vi "Main FPGA 6-axis Servo.vi"() -> ()   [LabVIEW 2014]
uses:
  <vilib>/Motion/MotorControl/_s/nism.encoder.config.ctl
  <vilib>/Motion/MotorControl/_s/nism.encoder.incremental.config.ctl
  <vilib>/Motion/MotorControl/_s/nism.incremental.indexCriteria.ctl
  <vilib>/Motion/MotorControl/_s/nism.pid.gains.fxp.18.ctl
  <vilib>/Motion/MotorControl/_s/nism.pi.v.outputRange.fxp.6.12.ctl
  <vilib>/Motion/MotorControl/_s/nism.mdo.splineData.ctl
  <vilib>/Motion/MotorControl/_s/nism.splineInterpolation.type.ctl
  <vilib>/Motion/SoftMotion/Synchronization/nism.softmotionScan.timerConfig.ctl
  <vilib>/Platform/TimedLoop/XDataNode/timing_clust.ctl
  <vilib>/Platform/TimedLoop/XDataNode/nitl_modes.ctl
  <vilib>/Platform/TimedLoop/XDataNode/wakeup.ctl
  <vilib>/Motion/MotorControl/_s/nism.digitalInputs.portA.ctl
  <vilib>/rvi/Emulation/niFpgaGetClockAttributes.vi
  <vilib>/rvi/Emulation/niFpgaSctlEmulationGetInTimedLoop.vi
  <vilib>/rvi/Emulation/niFpgaEmulationReportErrorSimple.vi
  Global FPGA 6-axis.vi
  <vilib>/Motion/MotorControl/_s/nism.interpretControlRegister.indexed.vi
  <vilib>/rvi/Emulation/niFpgaProcessEmulError.vi
  <vilib>/Motion/MotorControl/_s/nism.mdo.read.encoder.vi
  <vilib>/Motion/MotorControl/_s/nism.mdo.read.positionLoopSyncData.vi
  <vilib>/Motion/MotorControl/_s/nism.mdo.read.splineData.vi
  <vilib>/Motion/MotorControl/_s/nism.generateStatusRegister.indexed.vi
  <vilib>/rvi/eio/common/nirviEmuTemplateMethod_errors.vi
  <vilib>/rvi/Emulation/niFpgaCriticalErrorInLSC.vi
  <vilib>/Motion/MotorControl/_s/nism.splineInterpolation.fxp.3.index.vi
  <vilib>/Motion/MotorControl/_s/nism.pid.simple.fxp.index.2.vi
  <vilib>/Motion/MotorControl/_s/nism.mdo.handler.indexed.vi
  <vilib>/Motion/MotorControl/_s/nism.digitalFilter.indexed.vi
  <vilib>/Motion/MotorControl/_s/nism.interpretDIOControl.portA.multiple.vi
  <vilib>/Motion/MotorControl/_s/nism.generateDIOStatus.portA.indexed.2.vi
  <vilib>/Motion/SoftMotion/Synchronization/nism.rioScan.generateSyncScan.vi
  <vilib>/Motion/MotorControl/_s/nism.incremental.p.2.vi
  <vilib>/eio/EIONode/EIONode.xnode
  <vilib>/Platform/TimedLoop/XDataNode/XDataNode.xnode
  <vilib>/Motion/MotorControl/NI_SoftMotion_MotorControlIP.lvlib
  <vilib>/Platform/TimedLoop/XDataNode/XDNodeRunTimeDep.lvlib
  <vilib>/Motion/SoftMotion/Synchronization/NI_SoftMotion_Synchronization.lvlib
  <vilib>/rvi/Analysis/measure/butterworth/XNode/niFpgaButterworthFilter.xnode
panel:
  out "Interpolated Position":fxp<+/-,64,32>[](array[numeric])
  in  "Encoder Config (Manual)":T1={"active states"={"line a active high?"=FALSE, "line b active high?"=FALSE, "index active high?"=FALSE}, "index criteria"={"a"=FALSE, "b"=FALSE, "z"=FALSE}, "vel. filter coeffs."=[0, 0, 0]} caption="encoder config"
  in  "Velocity Filter Active?":bool
  in  "Reset Encoder 6":bool caption="reset"
  in  "Reset Encoder 5":bool caption="reset"
  in  "Reset Encoder 4":bool caption="reset"
  in  "Reset Encoder 3":bool caption="reset"
  out "position loop sync":T4
  out "spline":T5 {"spline type" items=["cubic b spline", "catmull-rom spline", "linear"]}
  in  "Reset Encoder 2":bool caption="reset"
  out "Velocity Feedback":i16[](array[numeric])
  out "pos. error":i16[](array[numeric])
  out "pos. error exceeded":bool[](array[boolean])
  in  "calls per sample (vel)":u16=2000 caption="calls per sample"
  in  "Limit Ranges":T7[](array[typedef])=[{"output low"=0.0, "output high"=0.0}, {"output low"=0.0, "output high"=0.0}, {"output low"=0.0, "output high"=0.0}, {"output low"=0.0, "output high"=0.0}, {"output low"=0.0, "output high"=0.0}, {"output low"=0.0, "output high"=0.0}]
  in  "Gains":T8[](array[typedef])=[{"kp"=0.0, "kd"=0.0, "ki"=0.0}, {"kp"=0.0, "kd"=0.0, "ki"=0.0}, {"kp"=0.0, "kd"=0.0, "ki"=0.0}, {"kp"=0.0, "kd"=0.0, "ki"=0.0}, {"kp"=0.0, "kd"=0.0, "ki"=0.0}, {"kp"=0.0, "kd"=0.0, "ki"=0.0}]
  out "AO Check":fxp<+/-,20,5>[](array[numeric])
  in  "AO Manual":fxp<+/-,20,5>[](array[numeric])=[0.0, 0.0, 0.0, 0.0, 0.0, 0.0]
  out "Position Feedback":i32[](array[numeric])
  in  "Reset Encoder 1":bool caption="reset"
  out "corrected period":u16
  in  "AO Disabled?":bool
  out "PID loop time (ticks)":u32
  in  "AO Override?":bool
  in  "position error limit":i16=10000
  in  "Encoder filter value (us) Manual":u16=10
  out "encoder config":T1
  out "Home Limits":bool[](array[boolean])
  out "Fwd Limits":bool[](array[boolean])
  out "Rev Limits":bool[](array[boolean])
  out "Drive Enable":bool[](array[boolean])
  in  "Enable value":bool
  in  "Drive Enable override?":bool
  in  "Sync Value":bool
  in  "Sync Enable override?":bool
  out "Sync is Fault":bool
  out "Sync is Locked":bool
  # "Synchronization Loop"
  # "Control Status Loop"
  # "Notes: \n1. This VI provides the communication interface between the NI SoftMotion Engine and the LabVIEW FPGA Module. You must compile this VI for a specific FPGA target before use. After compiling, run the VI before running any of the Express VI examples. For information on moving this example to another FPGA target, refer to ni.com/info and enter info code fpgaex.\n\n2. Only use the Reset Axis button if you are unable to communicate with the axis by any other means. This button resets the device state machine and other VIs to a known state. After resetting the axis, switch the NI Scan Engine from Active Mode to Configuration Mode, then back to Active Mode, before attempting to enable the axis."
  # "(These two buttons \nare for testing\npurposes.)"
  # "(These two buttons \nare for testing\npurposes.)"
  # "Position/PID Loop"
  # "Parameter Check"
  # "AO Debug"
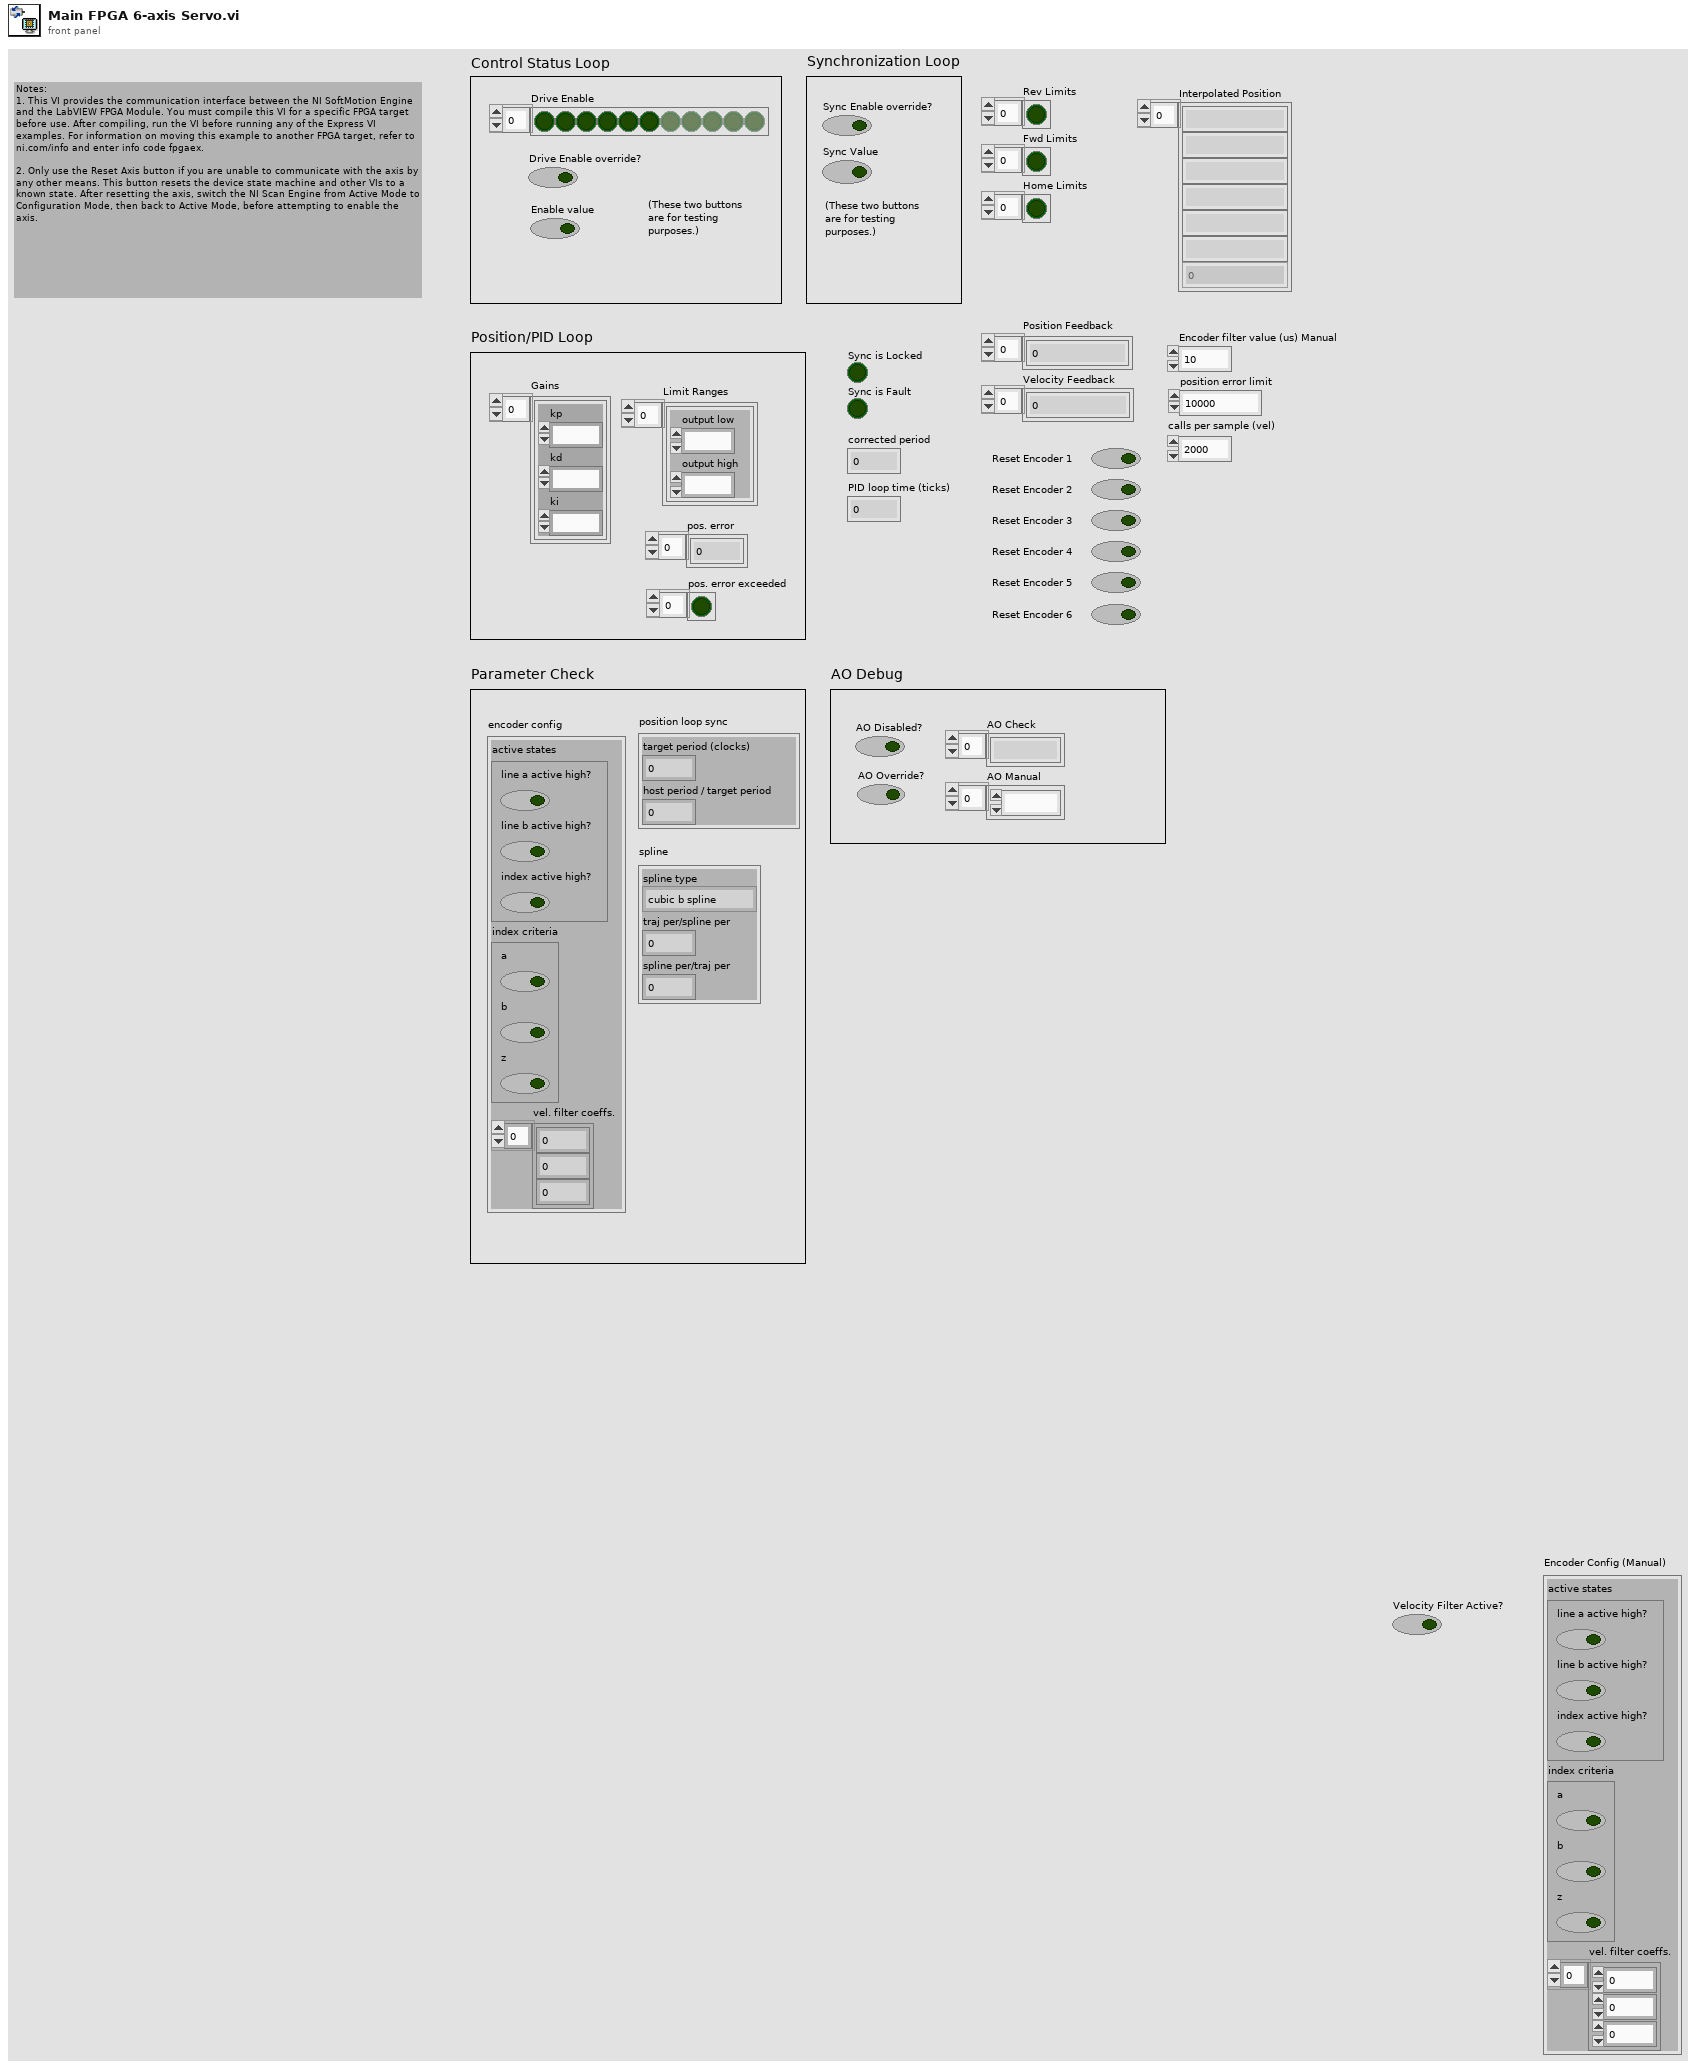
[diagram p1: front panel]
types:
  T1 = typedef "NI_SoftMotion_MotorControlIP.lvlib/nism.encoder.config.ctl" = cluster{"active states":T2, "index criteria":T3, "vel. filter coeffs.":i32[]}
  T2 = typedef "NI_SoftMotion_MotorControlIP.lvlib/nism.encoder.incremental.config.ctl" = cluster{"line a active high?":bool, "line b active high?":bool, "index active high?":bool}
  T3 = typedef "NI_SoftMotion_MotorControlIP.lvlib/nism.incremental.indexCriteria.ctl" = cluster{"a":bool, "b":bool, "z":bool}
  T4 = typedef "NI_SoftMotion_Synchronization.lvlib/nism.softmotionScan.timerConfig.ctl" = cluster{"target period (clocks)":u16, "host period / target period":u16}
  T5 = typedef "NI_SoftMotion_MotorControlIP.lvlib/nism.mdo.splineData.ctl" = cluster{"spline type":T6, "traj per/spline per":u16, "spline per/traj per":fxp<+,32,0>}
  T6 = typedef "NI_SoftMotion_MotorControlIP.lvlib/nism.splineInterpolation.type.ctl" = u16
  T7 = typedef "NI_SoftMotion_MotorControlIP.lvlib/nism.pi.v.outputRange.fxp.6.12.ctl" = cluster{"output low":fxp<+/-,18,6>, "output high":fxp<+/-,18,6>}
  T8 = typedef "NI_SoftMotion_MotorControlIP.lvlib/nism.pid.gains.fxp.18.ctl" = cluster{"kp":fxp<+,18,7>, "kd":fxp<+,18,7>, "ki":fxp<+,18,0>}
  T9 = typedef "XDNodeRunTimeDep.lvlib/timing_clust.ctl" = cluster{"Expected End [f-1]":u64, "Actual End [f-1]":u64, "Finished Late? [f-1]":bool, "Expected End [i-1]":u64, "Actual End [i-1]":u64, "Finished Late? [i-1]":bool, "Expected Start [i]":u64, "Actual Start [i]":u64, "Expected Start [f]":u64, "Actual Start [f]":u64, "Source Name":string, "Structure Name":string, "Period":i64, "Deadline":i64, "Offset":i64, "Start":i64, "Priority":i32, "Timeout":i32, "Mode":T10, "Wakeup Reason":T11, "Error":errorcluster, "Source Type":string, "Secondary Source Type":string, "Global End Time":u64, "Global Start Time":u64, "Frame Duration":u64, "Iteration Duration":u64, "Assigned CPU":i32, "I/O Scan Engine Mode":u32}
  T10 = typedef "XDNodeRunTimeDep.lvlib/nitl_modes.ctl" = enum32{"No Change", "Process missed periods, maintain original phase", "Discard missed periods, maintain original phase", "Process missed periods, ignore original phase", "Discard missed periods, ignore original phase"}
  T11 = typedef "XDNodeRunTimeDep.lvlib/wakeup.ctl" = enum32{"Normal", "Aborted", "Asynchronous wakeup", "Timing source error", "Timed loop error", "Timeout"}
  T12 = typedef "NI_SoftMotion_MotorControlIP.lvlib/nism.digitalInputs.portA.ctl" = cluster{"reverse limit":bool, "forward limit":bool, "home switch":bool, "digital input 0":bool, "digital input 1":bool, "digital input 2":bool, "digital input 3":bool}
  T13 = typedef "NI_SoftMotion_MotorControlIP.lvlib/nism.dio.portA.config.2.ctl" = cluster{"digital filter (us)":u16[], "safe state":T14[]}
  T14 = typedef "nism.safeStates.ctl" = enum8{"Low", "High", "No Change"}
  T15 = typedef "NI_SoftMotion_Synchronization.lvlib/nism.softmotionScan.timerControl.ctl" = cluster{"sm scan":bool, "sm scan count":u32, "sm scan enabled":bool}
  T16 = typedef "NI_SoftMotion_MotorControlIP.lvlib/nism.interpretControlRegister.stateTransition.ctl" = enum8{"Invalid", "Start --> Initializing", "Initializing --> Disabled", "Disabled --> Ready To Switch On", "Ready To Switch On --> Switched On", "Ready To Switch On --> Disable", "Switched On --> Operation Enable", "Switched On --> Ready To Switch On", "Switched On --> Disabled", "Operation Enable --> Switched On", "Operation Enable --> Ready To Switch On", "Operation Enable --> Disabled", "Fault --> Disabled", "Any --> Fault", "None"}
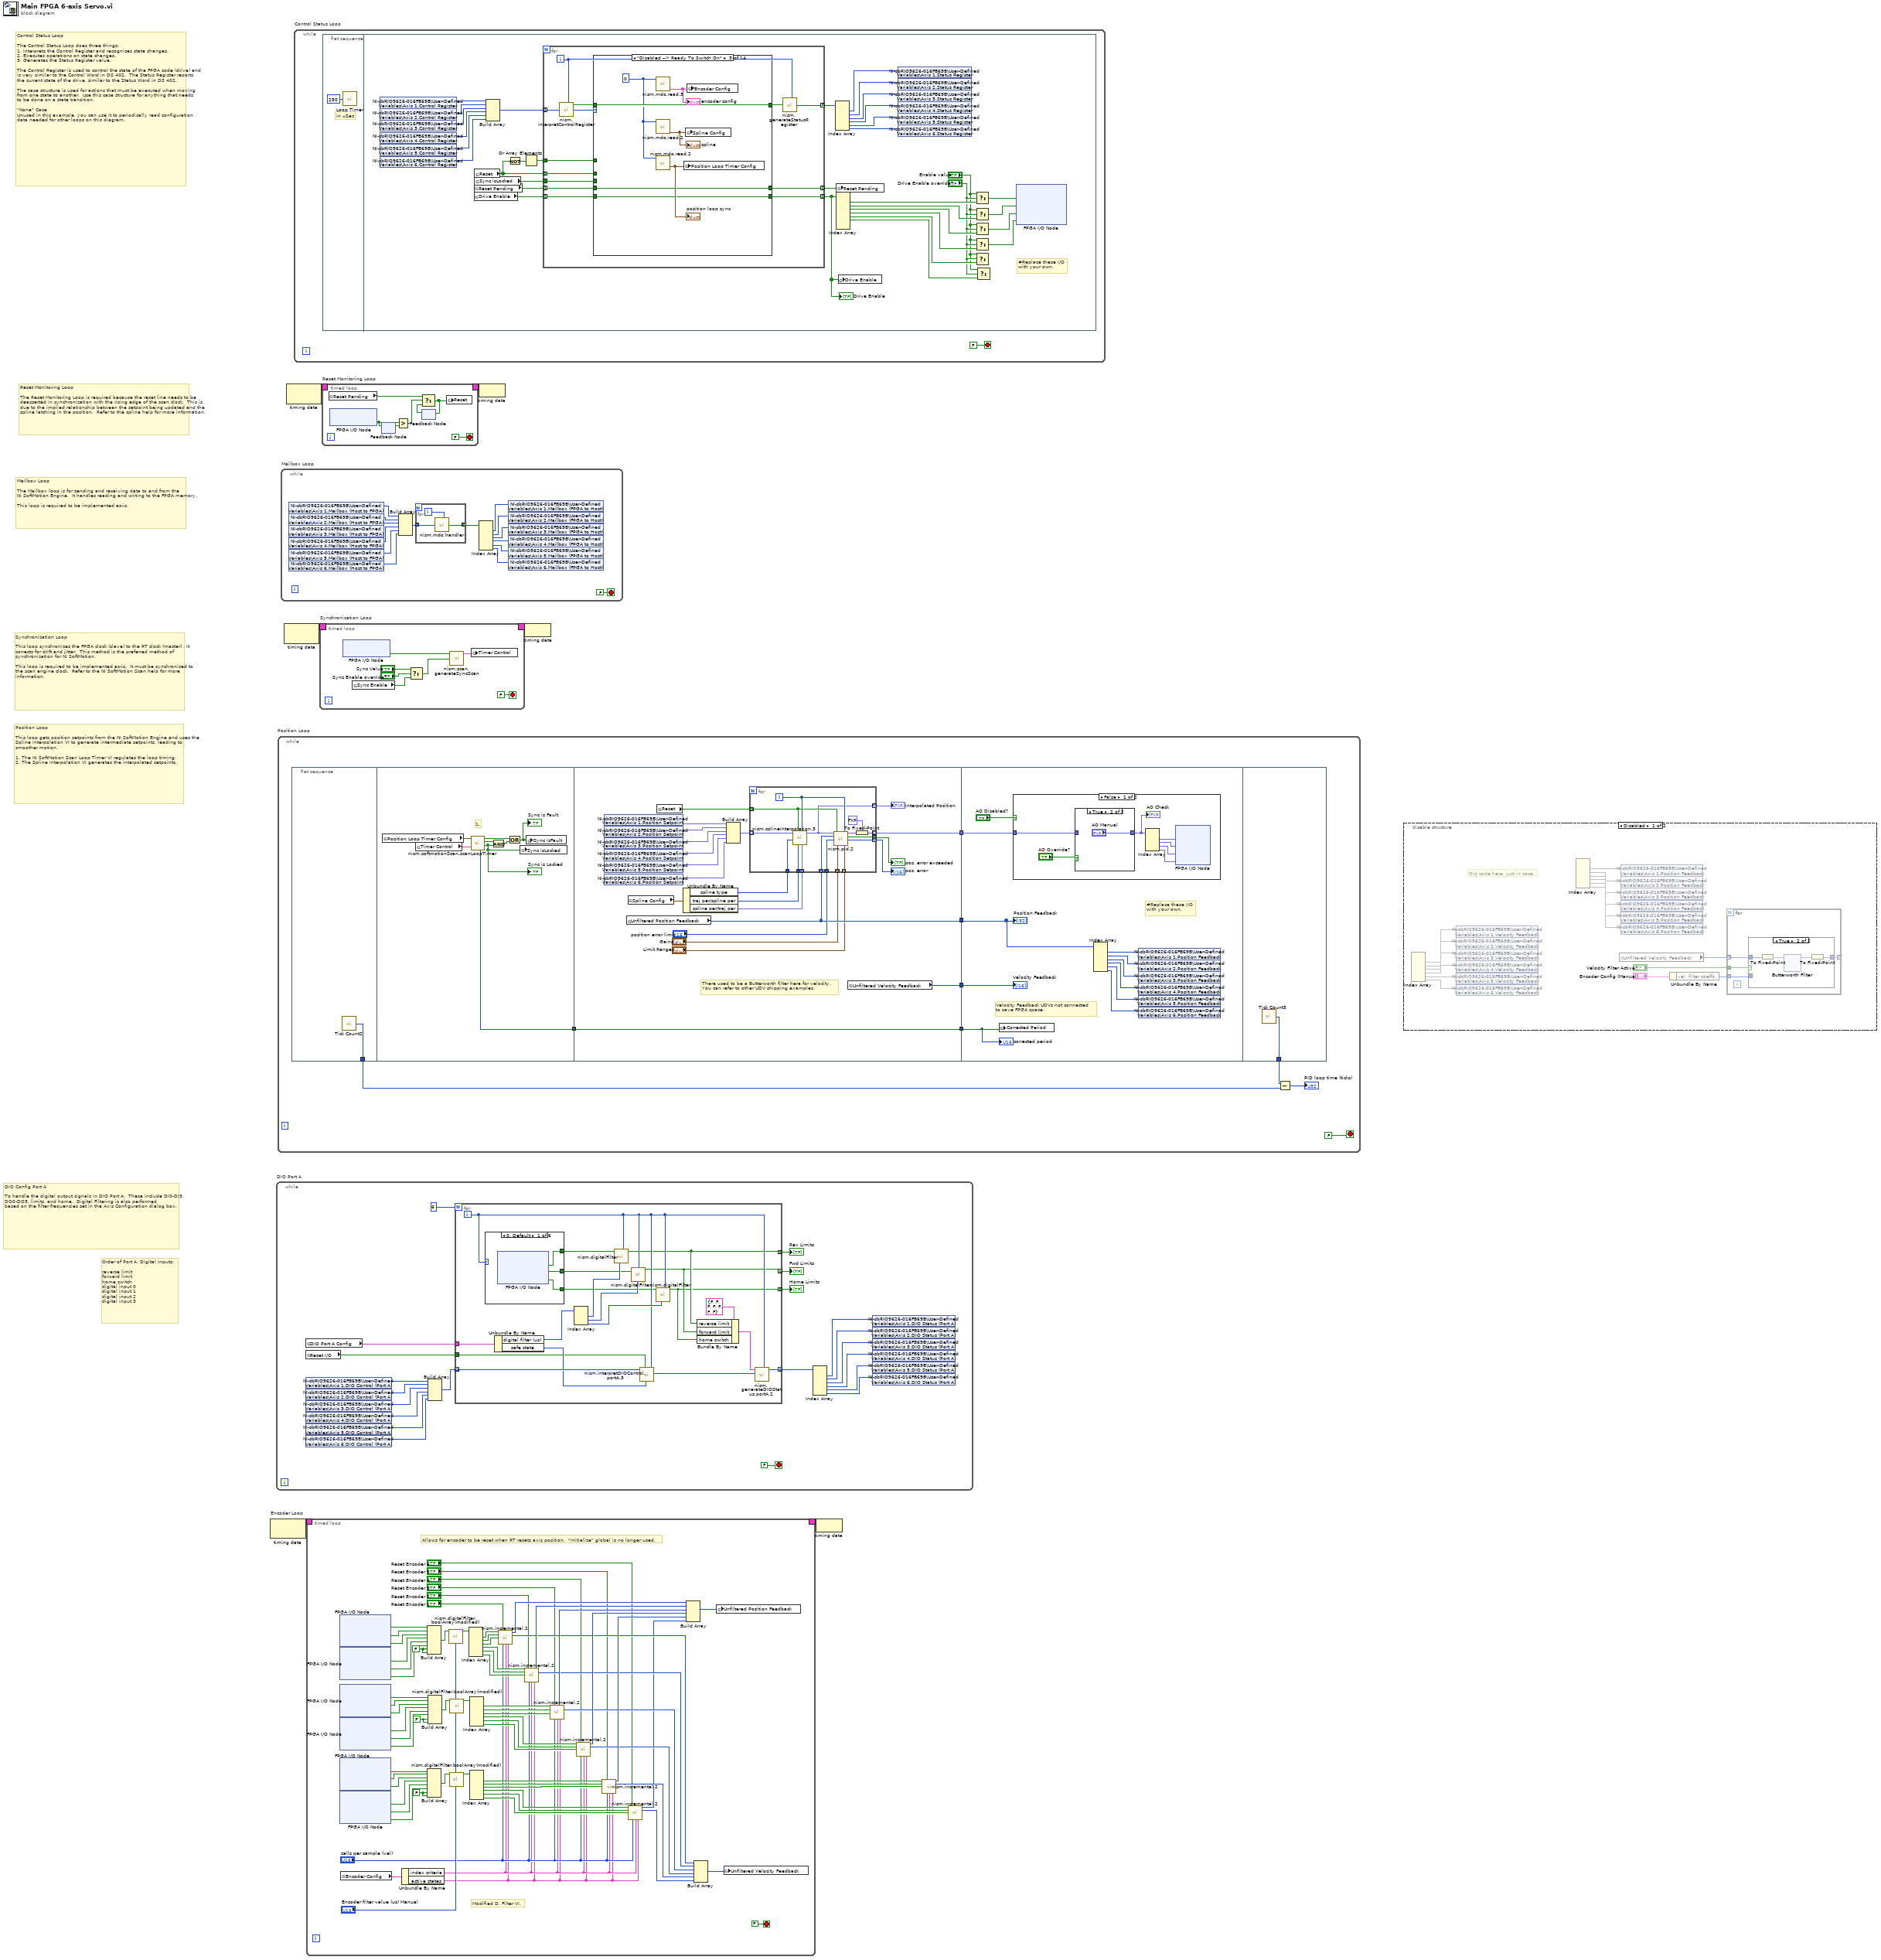
[diagram p0: block diagram]
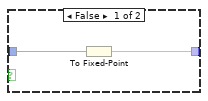
[diagram p2: hidden frame]
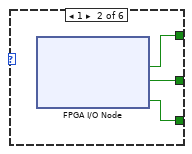
[diagram p4: hidden frame]
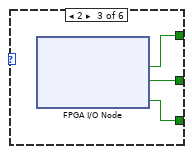
[diagram p5: hidden frame]
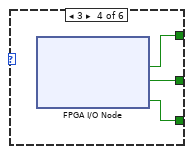
[diagram p6: hidden frame]
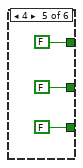
[diagram p7: hidden frame]
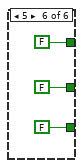
[diagram p8: hidden frame]
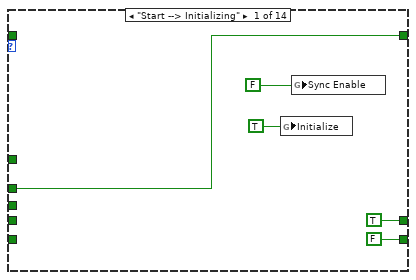
[diagram p11: hidden frame]
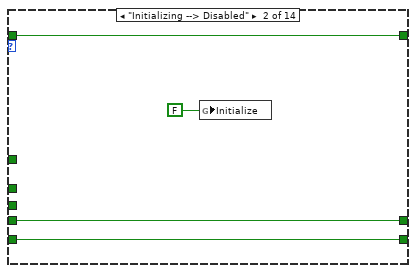
[diagram p12: hidden frame]
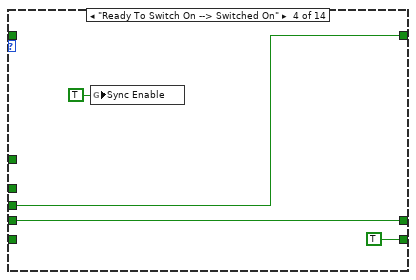
[diagram p13: hidden frame]
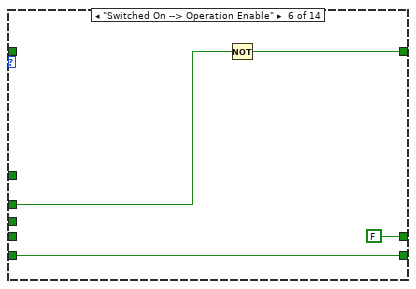
[diagram p15: hidden frame]
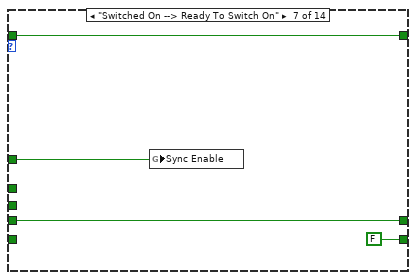
[diagram p16: hidden frame]
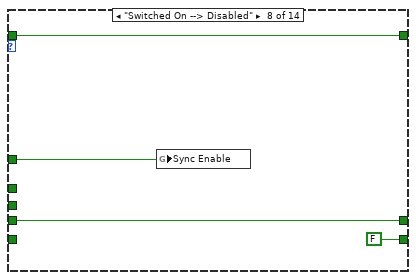
[diagram p17: hidden frame]
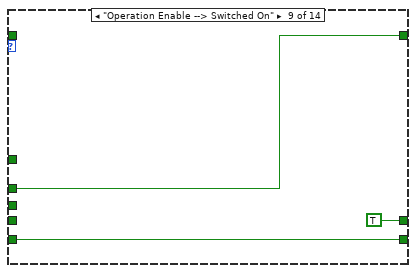
[diagram p18: hidden frame]
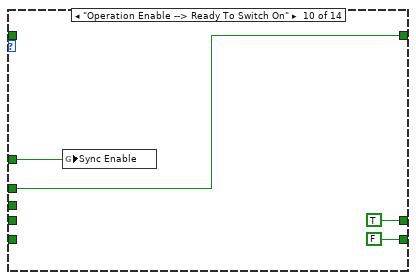
[diagram p19: hidden frame]
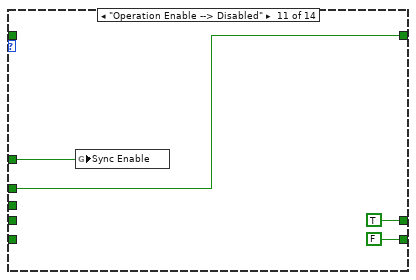
[diagram p20: hidden frame]
diagram:
  # "DIO Config Port A\n\nTo handle the digital output signals in DIO Port A.  These include DI0-DI3, DO0-DO3, limits, and home.  Digital Filtering is also performed\nbased on the filter frequencies set in the Axis Configuration dialog box."
  # "Order of Port A, Digital Inputs:\n\nreverse limit\nforward limit\nhome switch\ndigital input 0\ndigital input 1\ndigital input 2\ndigital input 3"
  # "Position Loop\n\nThis loop gets position setpoints from the NI SoftMotion Engine and uses the Spline Interpolation VI to generate intermediate setpoints, leading to smoother motion.\n\n1. The NI SoftMotion Scan Loop Timer VI regulates the loop timing. \n2. The Spline Interpolation VI generates the interpolated setpoints."
  # "Synchronization Loop\n\nThis loop synchronizes the FPGA clock (slave) to the RT clock (master).  It corrects for drift and jitter.  This method is the preferred method of synchronization for NI SoftMotion.\n\nThis loop is required to be implemented as-is.  It must be synchronized to the scan engine clock.  Refer to the NI SoftMotion Scan help for more information."
  # "Mailbox Loop\n\nThe Mailbox loop is for sending and receiving data to and from the \nNI SoftMotion Engine.  It handles reading and writing to the FPGA memory.\n\nThis loop is required to be implemented as-is."
  # "Reset Monitoring Loop\n\nThe Reset Monitoring Loop is required because the reset line needs to be deasserted in synchronization with the rising edge of the scan clock.  This is due to the implied relationship between the setpoint being updated and the spline latching in the position.  Refer to the spline help for more information."
  # "Control Status Loop\n\nThe Control Status Loop does three things:\n1. Interprets the Control Register and recognizes state changes.\n2. Executes operations on state changes.\n3. Generates the Status Register value.\n\nThe Control Register is used to control the state of the FPGA code (drive) and is very similar to the Control Word in DS 402.  The Status Register reports the current state of the drive, similar to the Status Word in DS 402.\n\nThe case structure is used for actions that must be executed when moving from one state to another.  Use this case structure for anything that needs to be done on a state transition.\n\n\"None\" Case\nUnused in this example, you can use it to periodically read configuration data needed for other loops on this diagram."
  n1 = node-c288() -> (w2:T9)  [unwired: 1 in]
  n2 = while "DIO Port A" {
    stop <- FALSE stop-if-true
    n3 = global read "Global FPGA 6-axis.vi" "DIO Port A Config"() -> (w26:T13)
    n4 = global read "Global FPGA 6-axis.vi" "Reset I/O"() -> (w25:bool)
    n5 = shared-variable "NI-sbRIO9626-016FB69B\\User-Defined Variables\\Axis 1.DIO Control (Port A)"() -> (w23:u32)  [unwired: 1 in, 1 out]
    n6 = shared-variable "NI-sbRIO9626-016FB69B\\User-Defined Variables\\Axis 2.DIO Control (Port A)"() -> (w22:u32)  [unwired: 1 in, 1 out]
    n7 = shared-variable "NI-sbRIO9626-016FB69B\\User-Defined Variables\\Axis 3.DIO Control (Port A)"() -> (w21:u32)  [unwired: 1 in, 1 out]
    n8 = shared-variable "NI-sbRIO9626-016FB69B\\User-Defined Variables\\Axis 4.DIO Control (Port A)"() -> (w20:u32)  [unwired: 1 in, 1 out]
    n9 = shared-variable "NI-sbRIO9626-016FB69B\\User-Defined Variables\\Axis 5.DIO Control (Port A)"() -> (w19:u32)  [unwired: 1 in, 1 out]
    n10 = shared-variable "NI-sbRIO9626-016FB69B\\User-Defined Variables\\Axis 6.DIO Control (Port A)"() -> (w8:u32)  [unwired: 1 in, 1 out]
    n11 = Build Array(w23, w22, w21, w20, w19, w8) -> (w18:u32[])
    n12 = for {
      N: 6 -> [_]
      tunnel: [w45] -> w12 mode=indexing
      tunnel: w18 -> [w44] mode=indexing
      tunnel: w26 -> [w41]
      tunnel: w25 -> [w39]
      tunnel: [w30] -> w11 mode=indexing
      tunnel: [w29] -> w10 mode=indexing
      tunnel: [w28] -> w9 mode=indexing
      i -> [w34]
      n13 = case shown="0, Default" w34 {
        tunnel: [w49 w52 w55 w58 FALSE ("RMC/DIO44") FALSE ("RMC/DIO44")] -> w33
        tunnel: [w47 w50 w53 w56 FALSE ("RMC/DIO61") FALSE ("RMC/DIO61")] -> w32
        tunnel: [w48 w51 w54 w57 FALSE ("RMC/DIO77") FALSE ("RMC/DIO77")] -> w31
        frame 0, Default {
          n14 = xnode "FPGA I/O Node"() -> ("RMC/DIO29"=w49:bool, "RMC/DIO93"=w48:bool, "RMC/DIO11"=w47:bool)  [unwired: 3 in, 3 out]
        }
        frame 1 {
          n15 = xnode "FPGA I/O Node"() -> ("RMC/DIO44"=w52:bool, "RMC/DIO77"=w51:bool, "RMC/DIO61"=w50:bool)  [unwired: 3 in, 3 out]
        }
        frame 2 {
          n16 = xnode "FPGA I/O Node"() -> ("RMC/DIO31"=w55:bool, "RMC/DIO95"=w54:bool, "RMC/DIO13"=w53:bool)  [unwired: 3 in, 3 out]
        }
        frame 3 {
          n17 = xnode "FPGA I/O Node"() -> ("RMC/DIO47"=w58:bool, "RMC/DIO46"=w57:bool, "RMC/DIO79"=w56:bool)  [unwired: 3 in, 3 out]
        }
        frame 4 {
        }
        frame 5 {
        }
      }
      n18 = Unbundle By Name(w41) -> ("digital filter (us)"=w35:u16[], "safe state"=w40:T14[])
      n19 = Index Array(array=w35) -> (element #1=w36:u16, element #2=w37:u16, element #3=w38:u16)  [unwired: 3 in]
      n20 = call-poly <vilib>:"nism.digitalFilter.vi"("index"=w34, "filter value (us)"=w36, "input signal"=w33) -> ("output signal"=w30:bool)  [unwired: 8 in]
      n21 = call-poly <vilib>:"nism.digitalFilter.vi"("index"=w34, "filter value (us)"=w37, "input signal"=w31) -> ("output signal"=w29:bool)  [unwired: 8 in]
      n22 = call-poly <vilib>:"nism.interpretDIOControl.portA.3.vi"("index"=w34, "safe state"=w40, "reset"=w39, "dio control(port a)"=w44) -> ("reset latches"=w46:u8)  [unwired: 6 in, 1 out]
      n23 = call-poly <vilib>:"nism.digitalFilter.vi"("index"=w34, "filter value (us)"=w38, "input signal"=w32) -> ("output signal"=w28:bool)  [unwired: 8 in]
      n24 = Bundle By Name(cluster=T12 {"reverse limit"=FALSE, "forward limit"=FALSE, "home switch"=FALSE, "digital input 0"=FALSE, "digital input 1"=FALSE, "digital input 2"=FALSE, "digital input 3"=FALSE} ("$(driveInterface.digitalInputs.shortName)"), "reverse limit"=w30, "forward limit"=w29, "home switch"=w28) -> (w42:T12)
      n25 = call-poly <vilib>:"nism.generateDIOStatus.portA.2.vi"("index"=w34, "reset latches"=w46, "digital inputs"=w42) -> ("dio status(port a)"=w45:u32)  [unwired: 8 in]
    }
    "Rev Limits" <- w11
    "Fwd Limits" <- w10
    "Home Limits" <- w9
    n26 = Index Array(array=w12) -> (element #1=w17:u32, element #2=w16:u32, element #3=w15:u32, element #4=w14:u32, element #5=w13:u32, element #6=w7:u32)  [unwired: 6 in]
    n27 = shared-variable "NI-sbRIO9626-016FB69B\\User-Defined Variables\\Axis 1.DIO Status (Port A)"(w17) -> ()  [unwired: 1 in, 1 out]
    n28 = shared-variable "NI-sbRIO9626-016FB69B\\User-Defined Variables\\Axis 2.DIO Status (Port A)"(w16) -> ()  [unwired: 1 in, 1 out]
    n29 = shared-variable "NI-sbRIO9626-016FB69B\\User-Defined Variables\\Axis 3.DIO Status (Port A)"(w15) -> ()  [unwired: 1 in, 1 out]
    n30 = shared-variable "NI-sbRIO9626-016FB69B\\User-Defined Variables\\Axis 4.DIO Status (Port A)"(w14) -> ()  [unwired: 1 in, 1 out]
    n31 = shared-variable "NI-sbRIO9626-016FB69B\\User-Defined Variables\\Axis 5.DIO Status (Port A)"(w13) -> ()  [unwired: 1 in, 1 out]
    n32 = shared-variable "NI-sbRIO9626-016FB69B\\User-Defined Variables\\Axis 6.DIO Status (Port A)"(w7) -> ()  [unwired: 1 in, 1 out]
  }
  n33 = while "Position Loop" {
    stop <- FALSE stop-if-true
    n34 = flat-sequence {
      tunnel: [w74] -> w68
      tunnel: [w75] -> w71
      tunnel: [w100] -> w72
      tunnel: w71 -> [w100]
      tunnel: [w90] -> w70
      tunnel: [w94] -> w66
      tunnel: [w84] -> w65
      tunnel: w72 -> [w131]
      tunnel: w70 -> [w121]
      tunnel: w66 -> [w130]
      tunnel: w65 -> [w128]
      tunnel: [w141] -> w69
      frame #0 {
        n35 = call "Tick Count2"() -> ("Tick Count(Ticks)"=w74:u32)
      }
      frame #1 {
        # "1."
        n36 = global read "Global FPGA 6-axis.vi" "Position Loop Timer Config"() -> (w77:T4)
        n37 = global read "Global FPGA 6-axis.vi" "Timer Control"() -> (w76:T15)
        n38 = call <vilib>:"nism.softmotionScan.scanLoopTimer.vi"("timer control"=w76, "timer config"=w77) -> ("scan running?"=w79:bool, "finished late?"=w81:bool, "fault occurred?"=w82:bool, "corrected period"=w75:u16)  [unwired: 5 in, 1 out]
        "Sync is Locked" <- w79
        n39 = Compound Arithmetic op=AND(w81, w79) -> (w80:bool)
        n40 = Compound Arithmetic op=OR(w82, w80) -> (w78:bool)
        "Sync is Fault" <- w78
        n41 = global write "Global FPGA 6-axis.vi" "Sync isLocked"(w79) -> ()
        n42 = global write "Global FPGA 6-axis.vi" "Sync isFault"(w78) -> ()
      }
      frame #2 {
        # "There used to be a Butterworth filter here for velocity.  \nYou can refer to other UDV shipping examples."
        n43 = shared-variable "NI-sbRIO9626-016FB69B\\User-Defined Variables\\Axis 1.Position Setpoint"() -> (w95:fxp<+/-,64,32>)  [unwired: 1 in, 1 out]
        n44 = shared-variable "NI-sbRIO9626-016FB69B\\User-Defined Variables\\Axis 2.Position Setpoint"() -> (w99:fxp<+/-,64,32>)  [unwired: 1 in, 1 out]
        n45 = shared-variable "NI-sbRIO9626-016FB69B\\User-Defined Variables\\Axis 3.Position Setpoint"() -> (w98:fxp<+/-,64,32>)  [unwired: 1 in, 1 out]
        n46 = shared-variable "NI-sbRIO9626-016FB69B\\User-Defined Variables\\Axis 4.Position Setpoint"() -> (w97:fxp<+/-,64,32>)  [unwired: 1 in, 1 out]
        n47 = shared-variable "NI-sbRIO9626-016FB69B\\User-Defined Variables\\Axis 5.Position Setpoint"() -> (w96:fxp<+/-,64,32>)  [unwired: 1 in, 1 out]
        n48 = shared-variable "NI-sbRIO9626-016FB69B\\User-Defined Variables\\Axis 6.Position Setpoint"() -> (w87:fxp<+/-,64,32>)  [unwired: 1 in, 1 out]
        n49 = global read "Global FPGA 6-axis.vi" "Unfiltered Position Feedback"() -> (w90:i32[])
        n50 = global read "Global FPGA 6-axis.vi" "Spline Config"() -> (w101:T5)
        n51 = global read "Global FPGA 6-axis.vi" "Reset"() -> (w92:bool[])
        n52 = Unbundle By Name(w101) -> ("spline type"=w104:T6, "traj per/spline per"=w103:u16, "spline per/traj per"=w102:fxp<+,32,0>)
        n53 = Build Array(w95, w99, w98, w97, w96, w87) -> (w93:fxp<+/-,64,32>[])
        n54 = for {
          tunnel: w104 -> [w120]
          tunnel: w103 -> [w119]
          tunnel: w102 -> [w118]
          tunnel: "Limit Ranges" -> [w117] mode=indexing
          tunnel: [w107] -> w94 mode=indexing
          tunnel: w93 -> [w116] mode=indexing
          tunnel: w92 -> [w114] mode=indexing
          tunnel: w90 -> [w113] mode=indexing
          tunnel: "position error limit" -> [w112]
          tunnel: [w111] -> w86 mode=indexing
          tunnel: [w110] -> w85 mode=indexing
          tunnel: "Gains" -> [w106] mode=indexing
          tunnel: [w105] -> w83 mode=indexing
          i -> [w115]
          n55 = call-poly <vilib>:"nism.splineInterpolation.3.vi"("1 / calls per sample"=w118, "index"=w115, "calls per sample"=w119, "reset"=w114, "spline type"=w120, "x"=w116) -> ("xi"=w105:fxp<+/-,64,32>)  [unwired: 4 in, 1 out]
          n56 = call-poly <vilib>:"nism.pid.2.vi"("position setpoint"=w105, "position feedback"=w113, "position error limit"=w112, "reset"=w114, "gains"=w106, "index"=w115, "output range"=w117) -> ("current setpoint"=w108:fxp<+/-,18,6>, "pos. error exceeded"=w111:bool, "position error"=w110:i16)  [unwired: 10 in]
          n57 = To Fixed-Point(fixed-point type=fxp<+/-,20,5> 0.0 ("AO 1"), number=w108) -> (fixed-point=w107:fxp<+/-,20,5>)
        }
        "pos. error exceeded" <- w86
        "pos. error" <- w85
        "Interpolated Position" <- w83
        n58 = global read "Global FPGA 6-axis.vi" "Unfiltered Velocity Feedback"() -> (w84:i16[])
      }
      frame #3 {
        # "Velocity Feedback UDVs not connected\nto save FPGA space."
        # "#Replace these I/O\nwith your own."
        n59 = global write "Global FPGA 6-axis.vi" "Corrected Period"(w131) -> ()
        n60 = case shown="False" "AO Disabled?" {
          tunnel: w130 -> [w137 _]
          frame False {
            n61 = case shown="True" "AO Override?" {
              tunnel: w137 -> [w139 _]
              tunnel: [w139 "AO Manual"] -> w136
              frame False {
              }
              frame True {
              }
            }
            "AO Check" <- w136
            n62 = Index Array(array=w136) -> (element #1=w135:fxp<+/-,20,5>, element #2=w134:fxp<+/-,20,5>, element #3=w133:fxp<+/-,20,5>, element #4=w132:fxp<+/-,20,5>)  [unwired: 4 in]
            n63 = xnode "FPGA I/O Node"("AO0"=w135, "AO1"=w134, "AO2"=w133, "AO3"=w132) -> ()  [unwired: 4 in, 4 out]
          }
          frame True {
          }
        }
        n64 = Index Array(array=w121) -> (element #1=w127:i32, element #2=w126:i32, element #3=w125:i32, element #4=w124:i32, element #5=w123:i32, element #6=w122:i32)  [unwired: 6 in]
        n65 = shared-variable "NI-sbRIO9626-016FB69B\\User-Defined Variables\\Axis 1.Position Feedback"(w127) -> ()  [unwired: 1 in, 1 out]
        n66 = shared-variable "NI-sbRIO9626-016FB69B\\User-Defined Variables\\Axis 2.Position Feedback"(w126) -> ()  [unwired: 1 in, 1 out]
        n67 = shared-variable "NI-sbRIO9626-016FB69B\\User-Defined Variables\\Axis 3.Position Feedback"(w125) -> ()  [unwired: 1 in, 1 out]
        n68 = shared-variable "NI-sbRIO9626-016FB69B\\User-Defined Variables\\Axis 4.Position Feedback"(w124) -> ()  [unwired: 1 in, 1 out]
        n69 = shared-variable "NI-sbRIO9626-016FB69B\\User-Defined Variables\\Axis 5.Position Feedback"(w123) -> ()  [unwired: 1 in, 1 out]
        n70 = shared-variable "NI-sbRIO9626-016FB69B\\User-Defined Variables\\Axis 6.Position Feedback"(w122) -> ()  [unwired: 1 in, 1 out]
        "corrected period" <- w131
        "Position Feedback" <- w121
        "Velocity Feedback" <- w128
      }
      frame #4 {
        n71 = call "Tick Count3"() -> ("Tick Count(Ticks)"=w141:u32)
      }
    }
    n72 = Subtract(x=w69, y=w68) -> (x-y=→"PID loop time (ticks)":u32)
  }
  n73 = while "Mailbox Loop" {
    stop <- FALSE stop-if-true
    n74 = shared-variable "NI-sbRIO9626-016FB69B\\User-Defined Variables\\Axis 1.Mailbox (Host to FPGA)"() -> (w153:u64)  [unwired: 1 in, 1 out]
    n75 = shared-variable "NI-sbRIO9626-016FB69B\\User-Defined Variables\\Axis 2.Mailbox (Host to FPGA)"() -> (w152:u64)  [unwired: 1 in, 1 out]
    n76 = shared-variable "NI-sbRIO9626-016FB69B\\User-Defined Variables\\Axis 3.Mailbox (Host to FPGA)"() -> (w151:u64)  [unwired: 1 in, 1 out]
    n77 = shared-variable "NI-sbRIO9626-016FB69B\\User-Defined Variables\\Axis 4.Mailbox (Host to FPGA)"() -> (w150:u64)  [unwired: 1 in, 1 out]
    n78 = shared-variable "NI-sbRIO9626-016FB69B\\User-Defined Variables\\Axis 5.Mailbox (Host to FPGA)"() -> (w149:u64)  [unwired: 1 in, 1 out]
    n79 = shared-variable "NI-sbRIO9626-016FB69B\\User-Defined Variables\\Axis 6.Mailbox (Host to FPGA)"() -> (w142:u64)  [unwired: 1 in, 1 out]
    n80 = Build Array(w153, w152, w151, w150, w149, w142) -> (w155:u64[])
    n81 = for {
      tunnel: w155 -> [w159] mode=indexing
      tunnel: [w158] -> w154 mode=indexing
      i -> [w157]
      n82 = call-poly <vilib>:"nism.mdo.handler.vi"("mbox (host to fpga)"=w159, "axis index"=w157) -> ("mbox (fpga to host)"=w158:u64)  [unwired: 7 in]
    }
    n83 = Index Array(array=w154) -> (element #1=w148:u64, element #2=w147:u64, element #3=w146:u64, element #4=w145:u64, element #5=w144:u64, element #6=w143:u64)  [unwired: 6 in]
    n84 = shared-variable "NI-sbRIO9626-016FB69B\\User-Defined Variables\\Axis 1.Mailbox (FPGA to Host)"(w148) -> ()  [unwired: 1 in, 1 out]
    n85 = shared-variable "NI-sbRIO9626-016FB69B\\User-Defined Variables\\Axis 2.Mailbox (FPGA to Host)"(w147) -> ()  [unwired: 1 in, 1 out]
    n86 = shared-variable "NI-sbRIO9626-016FB69B\\User-Defined Variables\\Axis 3.Mailbox (FPGA to Host)"(w146) -> ()  [unwired: 1 in, 1 out]
    n87 = shared-variable "NI-sbRIO9626-016FB69B\\User-Defined Variables\\Axis 4.Mailbox (FPGA to Host)"(w145) -> ()  [unwired: 1 in, 1 out]
    n88 = shared-variable "NI-sbRIO9626-016FB69B\\User-Defined Variables\\Axis 5.Mailbox (FPGA to Host)"(w144) -> ()  [unwired: 1 in, 1 out]
    n89 = shared-variable "NI-sbRIO9626-016FB69B\\User-Defined Variables\\Axis 6.Mailbox (FPGA to Host)"(w143) -> ()  [unwired: 1 in, 1 out]
  }
  n90 = node-c288() -> (w6:T9)  [unwired: 1 in]
  n91 = node-c288() -> (w4:T9)  [unwired: 1 in]
  n92 = while "Control Status Loop" {
    stop <- FALSE stop-if-true
    n93 = flat-sequence {
      frame #0 {
        # "in uSec"
        n94 = call "Loop Timer"("Count(uSec)"=u32 250) -> ()  [unwired: 1 out]
      }
      frame #1 {
        # "#Replace these I/O\nwith your own."
        n95 = shared-variable "NI-sbRIO9626-016FB69B\\User-Defined Variables\\Axis 1.Control Register"() -> (w185:u32)  [unwired: 1 in, 1 out]
        n96 = shared-variable "NI-sbRIO9626-016FB69B\\User-Defined Variables\\Axis 2.Control Register"() -> (w184:u32)  [unwired: 1 in, 1 out]
        n97 = shared-variable "NI-sbRIO9626-016FB69B\\User-Defined Variables\\Axis 3.Control Register"() -> (w183:u32)  [unwired: 1 in, 1 out]
        n98 = shared-variable "NI-sbRIO9626-016FB69B\\User-Defined Variables\\Axis 4.Control Register"() -> (w182:u32)  [unwired: 1 in, 1 out]
        n99 = shared-variable "NI-sbRIO9626-016FB69B\\User-Defined Variables\\Axis 5.Control Register"() -> (w181:u32)  [unwired: 1 in, 1 out]
        n100 = shared-variable "NI-sbRIO9626-016FB69B\\User-Defined Variables\\Axis 6.Control Register"() -> (w166:u32)  [unwired: 1 in, 1 out]
        n101 = global read "Global FPGA 6-axis.vi" "Reset Pending"() -> (w189:bool[])
        n102 = global read "Global FPGA 6-axis.vi" "Drive Enable"() -> (w188:bool[])
        n103 = global read "Global FPGA 6-axis.vi" "Reset"() -> (w190:bool[])
        n104 = global read "Global FPGA 6-axis.vi" "Sync isLocked"() -> (w195:bool)
        n105 = Build Array(w185, w184, w183, w182, w181, w166) -> (w194:u32[])
        n106 = Not(x=w190) -> (.not. x?=w192:bool[])
        n107 = Or Array Elements(Boolean array=w192) -> (logical OR=w191:bool)
        n108 = for {
          tunnel: w190 -> [w204] mode=indexing
          tunnel: w195 -> [w203]
          tunnel: w194 -> [w205] mode=indexing
          tunnel: [w202] -> w186 mode=indexing
          tunnel: [w201] -> w193 mode=indexing
          tunnel: [w200] -> w187 mode=indexing
          tunnel: w191 -> [w199]
          tunnel: w189 -> [w198] mode=indexing
          tunnel: w188 -> [w197] mode=indexing
          i -> [w206]
          n109 = call-poly <vilib>:"nism.interpretControlRegister.vi"("control register"=w205, "axis index"=w206) -> ("transition occurred"=w207:bool, "state transition"=w196:T16)  [unwired: 6 in]
          n110 = case shown="\"Disabled --> Ready To Switch On\"" w196 {
            tunnel: w207 -> [_ w217 w224 _ w231 _ w239 w243 _ _ _ _ w263 _]
            tunnel: [w213 w217 w224 w226 w231 w235 w239 w243 w245 w248 w252 w256 w262 _] -> w208
            tunnel: w204 -> [w213 _ _ _ _ w234 _ _ w245 w248 w252 w256 _ _]
            tunnel: w203 -> [_ _ _ w226 _ _ _ _ _ _ _ _ _ _]
            tunnel: [TRUE ("Write.Reset Pending") w216 w221 w225 w230 FALSE ("Write.Reset Pending") w236 w240 TRUE ("Write.Reset Pending") TRUE ("Write.Reset Pending") TRUE ("Write.Reset Pending") TRUE ("Write.Reset Pending") w260 w265] -> w201
            tunnel: [FALSE ("Write.Drive Enable") w215 w220 TRUE ("Write.Drive Enable") w229 w232 FALSE ("Write.Drive Enable") FALSE ("Write.Drive Enable") w244 FALSE ("Write.Drive Enable") FALSE ("Write.Drive Enable") FALSE ("Write.Drive Enable") w259 w264] -> w200
            tunnel: w199 -> [_ _ _ _ _ _ w237 w241 _ w247 w251 w255 w261 _]
            tunnel: w198 -> [_ w216 w221 w225 w230 _ w236 w240 _ _ _ _ w260 w265]
            tunnel: w197 -> [_ w215 w220 _ w229 w232 _ _ w244 _ _ _ w259 w264]
            frame "Start --> Initializing" {
              n111 = global write "Global FPGA 6-axis.vi" "Initialize"(TRUE ("Initialize")) -> ()
              n112 = global write "Global FPGA 6-axis.vi" "Sync Enable"(FALSE ("Sync Enable")) -> ()
            }
            frame "Initializing --> Disabled" {
              n113 = global write "Global FPGA 6-axis.vi" "Initialize"(FALSE ("Initialize")) -> ()
            }
            frame "Disabled --> Ready To Switch On" {
              w218 = 0 ("axis index")
              n114 = call-poly <vilib>:"nism.mdo.read.3.vi"("axis index"=w218) -> ("encoder config"=w219:T1)  [unwired: 10 in]
              "encoder config" <- w219
              n115 = call-poly <vilib>:"nism.mdo.read.2.vi"("axis index"=w218) -> ("spline"=w223:T5)  [unwired: 10 in]
              "spline" <- w223
              n116 = call-poly <vilib>:"nism.mdo.read.2.vi"("axis index"=w218) -> ("position loop sync"=w222:T4)  [unwired: 10 in]
              "position loop sync" <- w222
              n117 = global write "Global FPGA 6-axis.vi" "Position Loop Timer Config"(w222) -> ()
              n118 = global write "Global FPGA 6-axis.vi" "Spline Config"(w223) -> ()
              n119 = global write "Global FPGA 6-axis.vi" "Encoder Config"(w219) -> ()
            }
            frame "Ready To Switch On --> Switched On" {
              n120 = global write "Global FPGA 6-axis.vi" "Sync Enable"(TRUE ("Sync Enable")) -> ()
            }
            frame "Ready To Switch On --> Disable" {
            }
            frame "Switched On --> Operation Enable" {
              n121 = Not(x=w234) -> (.not. x?=w235:bool)
            }
            frame "Switched On --> Ready To Switch On" {
              n122 = global write "Global FPGA 6-axis.vi" "Sync Enable"(w237) -> ()
            }
            frame "Switched On --> Disabled" {
              n123 = global write "Global FPGA 6-axis.vi" "Sync Enable"(w241) -> ()
            }
            frame "Operation Enable --> Switched On" {
            }
            frame "Operation Enable --> Ready To Switch On" {
              n124 = global write "Global FPGA 6-axis.vi" "Sync Enable"(w247) -> ()
            }
            frame "Operation Enable --> Disabled" {
              n125 = global write "Global FPGA 6-axis.vi" "Sync Enable"(w251) -> ()
            }
            frame "Any --> Fault" {
              n126 = global write "Global FPGA 6-axis.vi" "Sync Enable"(w255) -> ()
            }
            frame "Fault --> Disabled" {
              # "wait one cycle for clear faults to have taken effect"
              n127 = global write "Global FPGA 6-axis.vi" "Sync Enable"(w261) -> ()
              n128 = Not(x=w263) -> (.not. x?=w262:bool)
            }
            frame "None", Default {
            }
          }
          n129 = call-poly <vilib>:"nism.generateStatusRegister.vi"("transition success"=w208, "axis index"=w206) -> ("status register"=w202:u32)  [unwired: 7 in]
        }
        "Drive Enable" <- w187
        n130 = Index Array(array=w186) -> (element #1=w180:u32, element #2=w179:u32, element #3=w178:u32, element #4=w177:u32, element #5=w176:u32, element #6=w165:u32)  [unwired: 6 in]
        n131 = global write "Global FPGA 6-axis.vi" "Reset Pending"(w193) -> ()
        n132 = Index Array(array=w187) -> (element #1=w175:bool, element #2=w174:bool, element #3=w173:bool, element #4=w172:bool, element #5=w171:bool, element #6=w164:bool)  [unwired: 8 in, 2 out]
        n133 = global write "Global FPGA 6-axis.vi" "Drive Enable"(w187) -> ()
        n134 = shared-variable "NI-sbRIO9626-016FB69B\\User-Defined Variables\\Axis 1.Status Register"(w180) -> ()  [unwired: 1 in, 1 out]
        n135 = shared-variable "NI-sbRIO9626-016FB69B\\User-Defined Variables\\Axis 2.Status Register"(w179) -> ()  [unwired: 1 in, 1 out]
        n136 = shared-variable "NI-sbRIO9626-016FB69B\\User-Defined Variables\\Axis 3.Status Register"(w178) -> ()  [unwired: 1 in, 1 out]
        n137 = shared-variable "NI-sbRIO9626-016FB69B\\User-Defined Variables\\Axis 4.Status Register"(w177) -> ()  [unwired: 1 in, 1 out]
        n138 = shared-variable "NI-sbRIO9626-016FB69B\\User-Defined Variables\\Axis 5.Status Register"(w176) -> ()  [unwired: 1 in, 1 out]
        n139 = shared-variable "NI-sbRIO9626-016FB69B\\User-Defined Variables\\Axis 6.Status Register"(w165) -> ()  [unwired: 1 in, 1 out]
        n140 = Select(t="Enable value", s="Drive Enable override?", f=w175) -> (s? t:f=w170:bool)
        n141 = Select(t="Enable value", s="Drive Enable override?", f=w174) -> (s? t:f=w169:bool)
        n142 = Select(t="Enable value", s="Drive Enable override?", f=w173) -> (s? t:f=w168:bool)
        n143 = Select(t="Enable value", s="Drive Enable override?", f=w172) -> (s? t:f=w167:bool)
        n144 = Select(t="Enable value", s="Drive Enable override?", f=w171) -> ()  [unwired: 1 out]
        n145 = Select(t="Enable value", s="Drive Enable override?", f=w164) -> ()  [unwired: 1 out]
        n146 = xnode "FPGA I/O Node"("RMC/DIO28"=w170, "RMC/DIO12"=w169, "RMC/DIO30"=w168, "RMC/DIO14"=w167) -> ()  [unwired: 4 in, 4 out]
      }
    }
  }
  n147 = timed-loop "Encoder Loop" {
    timing: w2 -> [_]
    timing-out: [_] -> w1
    stop <- FALSE stop-if-true
    w293 = FALSE ("element")
    w294 = FALSE ("element")
    w310 = FALSE ("element")
    # "Allows for encoder to be reset when RT resets axis position.  \"Initialize\" global is no longer used."
    # "Modified D. Filter VI."
    n148 = xnode "FPGA I/O Node"() -> ("RMC/DIO60"=w334:bool, "RMC/DIO42"=w335:bool, "RMC/DIO75"=w333:bool)  [unwired: 3 in, 3 out]
    n149 = xnode "FPGA I/O Node"() -> ("RMC/DIO59"=w315:bool, "RMC/DIO92"=w314:bool, "RMC/DIO10"=w313:bool)  [unwired: 3 in, 3 out]
    n150 = xnode "FPGA I/O Node"() -> ("RMC/DIO74"=w306:bool, "RMC/DIO27"=w305:bool, "RMC/DIO91"=w304:bool)  [unwired: 3 in, 3 out]
    n151 = xnode "FPGA I/O Node"() -> ("RMC/DIO9"=w303:bool, "RMC/DIO41"=w302:bool, "RMC/DIO26"=w301:bool)  [unwired: 3 in, 3 out]
    n152 = xnode "FPGA I/O Node"() -> ("RMC/DIO58"=w287:bool, "RMC/DIO40"=w288:bool, "RMC/DIO73"=w289:bool)  [unwired: 3 in, 3 out]
    n153 = xnode "FPGA I/O Node"() -> ("RMC/DIO57"=w290:bool, "RMC/DIO90"=w291:bool, "RMC/DIO8"=w292:bool)  [unwired: 3 in, 3 out]
    n154 = global read "Global FPGA 6-axis.vi" "Encoder Config"() -> (w270:T1)
    n155 = Unbundle By Name(w270) -> ("index criteria"=w273:T3, "active states"=w272:T2)
    n156 = Build Array(w334, w335, w333, w315, w314, w313, w310, w310) -> (w332:bool[])
    n157 = Build Array(w287, w288, w289, w290, w291, w292, w293, w293) -> (w286:bool[])
    n158 = Build Array(w306, w305, w304, w303, w302, w301, w294, w294) -> (w311:bool[])
    n159 = call "nism.digitalFilter.boolArray(modified).vi"("filter value (us)"="Encoder filter value (us) Manual", "input signal"=w332) -> ("output signal"=w331:bool[])  [unwired: 9 in]
    n160 = call "nism.digitalFilter.boolArray(modified).vi"("filter value (us)"="Encoder filter value (us) Manual", "input signal"=w286) -> ("output signal"=w285:bool[])  [unwired: 9 in]
    n161 = call "nism.digitalFilter.boolArray(modified).vi"("filter value (us)"="Encoder filter value (us) Manual", "input signal"=w311) -> ("output signal"=w312:bool[])  [unwired: 9 in]
    n162 = Index Array(array=w331) -> (element #1=w330:bool, element #2=w329:bool, element #3=w328:bool, element #4=w309:bool, element #5=w308:bool, element #6=w307:bool)  [unwired: 6 in]
    n163 = Index Array(array=w285) -> (element #1=w284:bool, element #2=w283:bool, element #3=w282:bool, element #4=w279:bool, element #5=w278:bool, element #6=w277:bool)  [unwired: 6 in]
    n164 = Index Array(array=w312) -> (element #1=w300:bool, element #2=w299:bool, element #3=w298:bool, element #4=w297:bool, element #5=w296:bool, element #6=w295:bool)  [unwired: 6 in]
    n165 = call-poly <vilib>:"nism.incremental.2.vi"("a phase"=w330, "reset"="Reset Encoder 1", "b phase"=w329, "z phase"=w328, "calls per sample"="calls per sample (vel)", "index criteria"=w273, "active states"=w272) -> ("encoder position"=w327:i32, "velocity"=w320:i16)  [unwired: 5 in, 2 out]
    n166 = call-poly <vilib>:"nism.incremental.2.vi"("a phase"=w309, "reset"="Reset Encoder 2", "b phase"=w308, "z phase"=w307, "calls per sample"="calls per sample (vel)", "index criteria"=w273, "active states"=w272) -> ("encoder position"=w326:i32, "velocity"=w319:i16)  [unwired: 5 in, 2 out]
    n167 = call-poly <vilib>:"nism.incremental.2.vi"("a phase"=w300, "reset"="Reset Encoder 3", "b phase"=w299, "z phase"=w298, "calls per sample"="calls per sample (vel)", "index criteria"=w273, "active states"=w272) -> ("encoder position"=w325:i32, "velocity"=w318:i16)  [unwired: 5 in, 2 out]
    n168 = call-poly <vilib>:"nism.incremental.2.vi"("a phase"=w297, "reset"="Reset Encoder 4", "b phase"=w296, "z phase"=w295, "calls per sample"="calls per sample (vel)", "index criteria"=w273, "active states"=w272) -> ("encoder position"=w324:i32, "velocity"=w317:i16)  [unwired: 5 in, 2 out]
    n169 = call-poly <vilib>:"nism.incremental.2.vi"("a phase"=w284, "reset"="Reset Encoder 5", "b phase"=w283, "z phase"=w282, "calls per sample"="calls per sample (vel)", "index criteria"=w273, "active states"=w272) -> ("encoder position"=w323:i32, "velocity"=w316:i16)  [unwired: 5 in, 2 out]
    n170 = call-poly <vilib>:"nism.incremental.2.vi"("a phase"=w279, "reset"="Reset Encoder 6", "b phase"=w278, "z phase"=w277, "calls per sample"="calls per sample (vel)", "index criteria"=w273, "active states"=w272) -> ("encoder position"=w276:i32, "velocity"=w275:i16)  [unwired: 5 in, 2 out]
    n171 = Build Array(w327, w326, w325, w324, w323, w276) -> (w322:i32[])
    n172 = Build Array(w320, w319, w318, w317, w316, w275) -> (w321:i16[])
    n173 = global write "Global FPGA 6-axis.vi" "Unfiltered Position Feedback"(w322) -> ()
    n174 = global write "Global FPGA 6-axis.vi" "Unfiltered Velocity Feedback"(w321) -> ()
  }
  n175 = timed-loop "Synchronization Loop" {
    timing: w6 -> [_]
    timing-out: [_] -> w5
    stop <- FALSE stop-if-true
    n176 = xnode "FPGA I/O Node"() -> ("Scan Clock"=w343:bool)  [unwired: 1 in, 1 out]
    n177 = global read "Global FPGA 6-axis.vi" "Sync Enable"() -> (w342:bool)
    n178 = Select(t="Sync Value", s="Sync Enable override?", f=w342) -> (s? t:f=w339:bool)
    n179 = call-poly <vilib>:"nism.scan.generateSyncScan.vi"("scan enable?"=w339, "scan clock"=w343) -> ("timer control"=w344:T15)  [unwired: 3 in]
    n180 = global write "Global FPGA 6-axis.vi" "Timer Control"(w344) -> ()
  }
  n181 = timed-loop "Reset Monitoring Loop" {
    timing: w4 -> [_]
    timing-out: [_] -> w3
    stop <- FALSE stop-if-true
    n182 = global read "Global FPGA 6-axis.vi" "Reset Pending"() -> (w350:bool[])
    n183 = xnode "FPGA I/O Node"() -> ("Scan Clock"=w349:bool)  [unwired: 1 in, 1 out]
    n184 = feedback-in #1(w349) -> ()
    n185 = feedback #1() -> (w348:bool)  [unwired: 1 in]
    n186 = Greater?(x=w349, y=w348) -> (0:w354:bool)
    n187 = feedback #2() -> (w353:bool[])  [unwired: 1 in]
    n188 = Select(t=w350, s=w354, f=w353) -> (s? t:f=w351:bool[])
    n189 = feedback-in #2(w351) -> ()
    n190 = global write "Global FPGA 6-axis.vi" "Reset"(w351) -> ()
  }
  n191 = node-c288(w3) -> ()
  n192 = node-c288(w5) -> ()
  n193 = node-c288(w1) -> ()
  n194 = disable-structure shown="Disabled" {
    frame Disabled {
      # "Old code here, just in case."
      n195 = Index Array() -> (element #1=w367, element #2=w368, element #3=w369, element #4=w370, element #5=w371, element #6=w372)  [unwired: 7 in]
      n196 = shared-variable "NI-sbRIO9626-016FB69B\\User-Defined Variables\\Axis 1.Velocity Feedback"(w367) -> ()  [unwired: 1 in, 1 out]
      n197 = shared-variable "NI-sbRIO9626-016FB69B\\User-Defined Variables\\Axis 2.Velocity Feedback"(w368) -> ()  [unwired: 1 in, 1 out]
      n198 = shared-variable "NI-sbRIO9626-016FB69B\\User-Defined Variables\\Axis 3.Velocity Feedback"(w369) -> ()  [unwired: 1 in, 1 out]
      n199 = shared-variable "NI-sbRIO9626-016FB69B\\User-Defined Variables\\Axis 4.Velocity Feedback"(w370) -> ()  [unwired: 1 in, 1 out]
      n200 = shared-variable "NI-sbRIO9626-016FB69B\\User-Defined Variables\\Axis 5.Velocity Feedback"(w371) -> ()  [unwired: 1 in, 1 out]
      n201 = shared-variable "NI-sbRIO9626-016FB69B\\User-Defined Variables\\Axis 6.Velocity Feedback"(w372) -> ()  [unwired: 1 in, 1 out]
      n202 = Index Array() -> (element #1=w357, element #2=w358, element #3=w359, element #4=w360, element #5=w361, element #6=w362)  [unwired: 7 in]
      n203 = global read "Global FPGA 6-axis.vi" "Unfiltered Velocity Feedback"() -> (w365:i16[])
      n204 = shared-variable "NI-sbRIO9626-016FB69B\\User-Defined Variables\\Axis 1.Position Feedback"(w357) -> ()  [unwired: 1 in, 1 out]
      n205 = shared-variable "NI-sbRIO9626-016FB69B\\User-Defined Variables\\Axis 2.Position Feedback"(w358) -> ()  [unwired: 1 in, 1 out]
      n206 = shared-variable "NI-sbRIO9626-016FB69B\\User-Defined Variables\\Axis 3.Position Feedback"(w359) -> ()  [unwired: 1 in, 1 out]
      n207 = shared-variable "NI-sbRIO9626-016FB69B\\User-Defined Variables\\Axis 4.Position Feedback"(w360) -> ()  [unwired: 1 in, 1 out]
      n208 = shared-variable "NI-sbRIO9626-016FB69B\\User-Defined Variables\\Axis 5.Position Feedback"(w361) -> ()  [unwired: 1 in, 1 out]
      n209 = shared-variable "NI-sbRIO9626-016FB69B\\User-Defined Variables\\Axis 6.Position Feedback"(w362) -> ()  [unwired: 1 in, 1 out]
      n210 = Unbundle By Name("Encoder Config (Manual)") -> ("vel. filter coeffs."=w366:i32[])
      n211 = for {
        tunnel: "Velocity Filter Active?" -> [w376]
        tunnel: w366 -> [w375] mode=indexing
        tunnel: w365 -> [w374] mode=indexing
        tunnel: [w373] -> _ mode=indexing
        n212 = case shown="True" w376 {
          tunnel: w374 -> [w378 w382]
          tunnel: w375 -> [_ _]
          tunnel: [w377 w380] -> w373
          frame False {
            n213 = To Fixed-Point(number=w378) -> (fixed-point=w377:fxp<+/-,64,32>)  [unwired: 1 in]
          }
          frame True {
            n214 = To Fixed-Point(number=w382) -> (fixed-point=w381:fxp<+/-,16,16>)  [unwired: 1 in]
            n215 = xnode "Butterworth Filter"("input data"=w381) -> ("output data"=w379:fxp<+/-,16,16>)  [unwired: 2 in, 1 out]
            n216 = To Fixed-Point(number=w379) -> (fixed-point=w380:fxp<+/-,64,32>)  [unwired: 1 in]
          }
        }
      }
    }
    frame Enabled {
    }
  }
